vi "serialRead_p.vi"(0 "baseAdderess":u32=3774873600 format="%.0x", 1 "serialBoard":u16(ring) items=["DEVIL", "M17"], 2 "subID1 (0)":u32 format="%.0x", 3 "subID2 (0)":u32, 4 "controlCharacter (0)":u16 format="%.0x", 5 "timeOut [ms] (1000)":i32=1000) -> (6 "string read":string, 7 "errorCode":cdb format="%.2f", 8 "errorSpec":i32)   [LabVIEW 2010]
doc: "reads the content of the input buffer of the serial port indicated by \"subID1\" and \"subID2\". The read process ends when the buffer is empty or a control character has been encountered (depending on the \"controlCharacter\" value and how the serial channel has been inited.\nWARNING: remember to setup the serial channel before running this routine using:\n1. \"serialInitialize.vi\" for hardware setup;\n2. \"serialConfigure\" for software setup."
uses:
  <userlib>/libcommon_serial/libcommon_serial.lvlib
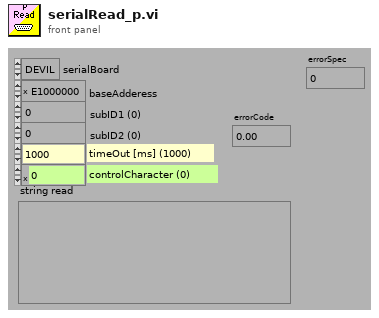
[diagram p1: front panel]
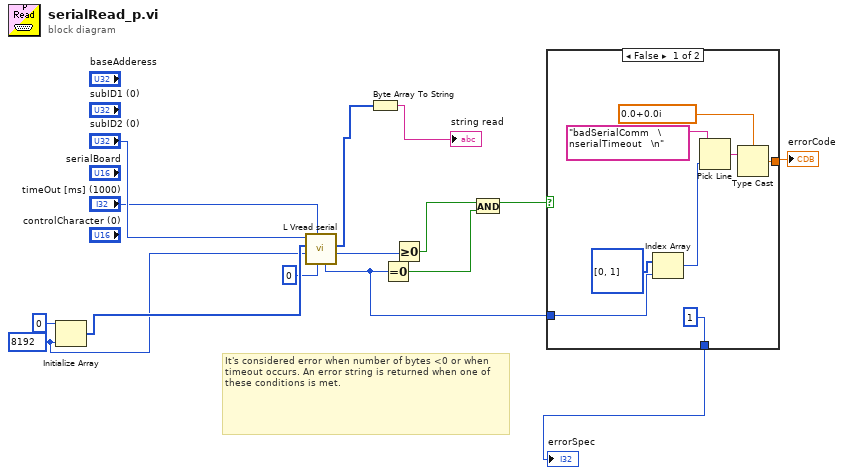
[diagram p0: block diagram]
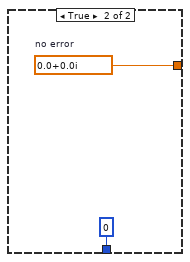
[diagram p2: hidden frame]
diagram:
  w10 = 8192 ("dimension size")
  # "It's considered error when number of bytes <0 or when timeout occurs. An error string is returned when one of these conditions is met."
  n1 = Initialize Array(u8 0 ("element"), w10) -> (w11:u8[])
  n2 = call <userlib>:"L Vread serial.vi"("timoccur"=0, "timeo"="timeOut [ms] (1000)", "bsize"=w10, "buf"=w11, "resourceId"="subID2 (0)") -> ("byte read"=w7:i32, "buf out"=w9:u8[], "timoccur out"=w2:i32)  [unwired: 3 in, 1 out]
  n3 = Byte Array To String(unsigned byte array=w9) -> (string=→"string read":string)
  n4 = Equal To 0?(x=w2) -> (x = 0?=w3:bool)
  n5 = Greater Or Equal To 0?(x=w7) -> (x >= 0?=w6:bool)
  n6 = And(x=w6, y=w3) -> (x .and. y?=w4:bool)
  n7 = case shown="False" w4 {
    tunnel: [w20 w25] -> w15
    tunnel: w2 -> [w17 _]
    tunnel: [1 0] -> w1
    frame False {
      n8 = Index Array(array=i32[] [0, 1], index=w17) -> (element=w19:i32)
      n9 = Pick Line(multi-line string="badSerialComm   \nserialTimeout   \n", line index=w19) -> (output string=w22:string)  [unwired: 1 in]
      n10 = Type Cast(type=cdb 0.0+0.0i, x=w22) -> (*(type *) &x=w20:cdb)
    }
    frame True {
      w25 = cdb 0.0+0.0i  # no error
    }
  }
  "errorCode" <- w15
  "errorSpec" <- w1
